vi "Create.vi"(5 "Project Inspector in":refnum<class "Project Inspector.lvclass">, 8 "error in (no error)":errorcluster, 11 "Project":refnum<vi>) -> (0 "error out":errorcluster, 3 "Project Inspector":refnum<class "Project Inspector.lvclass">)   [LabVIEW 2017, in "Cobertura.lvlib" / "Project Inspector.lvclass"]
uses:
  Project Inspector.lvclass
  Project Inspector.lvclass/Project Inspector.ctl
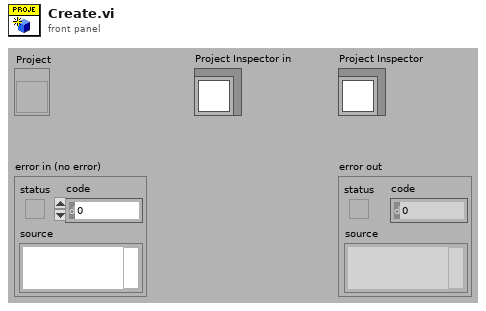
[diagram p1: front panel]
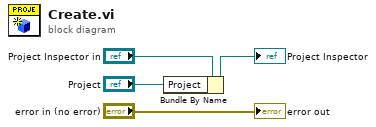
[diagram p0: block diagram]
diagram:
  n1 = Bundle By Name(cluster="Project Inspector in", "Project"="Project") -> (→"Project Inspector":refnum<class "Project Inspector.lvclass">)
  "error out" <- "error in (no error)"
